vi "PSA E4440A Set and Read Marker X and Y Values.vi"(0 "VISA resource name":refnum<visa-resource-name>, 1 "Marker Type (1: Position)":u16(ring)=1 items=["Off", "Position", "Delta", "Band", "Span Pair"], 2 "Readout (0: Frequency)":u16(ring) items=["Frequency", "Time", "Inverse Time", "Period"], 5 "Active Marker (1: Marker1)":u16(ring)=1 items=["Marker1"=1, "Marker2"=2, "Marker3"=3, "Marker4"=4], 9 "Zero Span":bool, 11 "error in (no error)":errorcluster, 12 "Span [Hz]":dbl=5000000.0 format="%.3p", 13 "Center Frequency (Hz)":dbl=2000000000.0) -> (4 "VISA resource name out":refnum<visa-resource-name>, 6 "Marker X Position (Hz)":dbl, 8 "Y Amplitude (dBm)":dbl, 15 "error out":errorcluster)   [LabVIEW 2015]
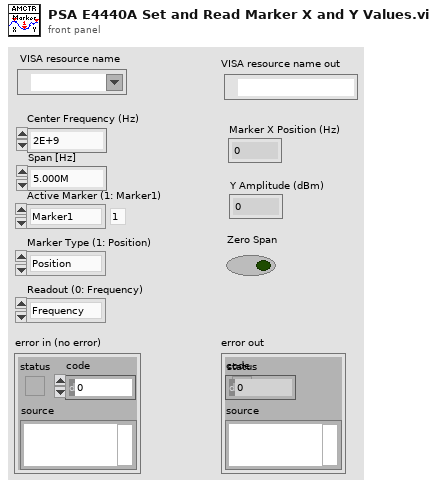
[diagram p1: front panel]
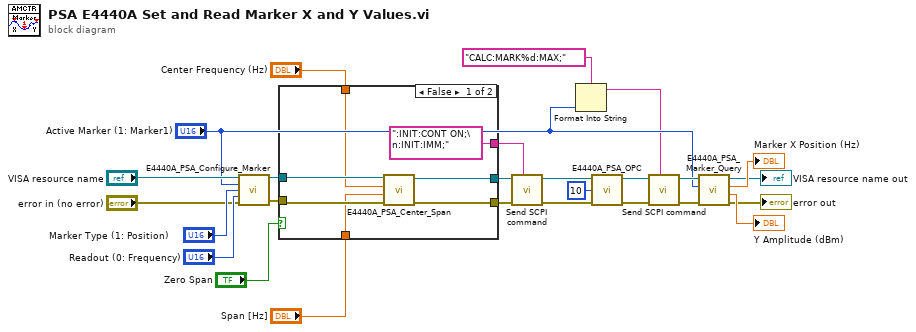
[diagram p0: block diagram]
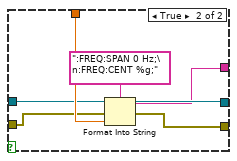
[diagram p2: hidden frame]
diagram:
  n1 = call "E4440A_PSA_Configure_Marker.vi"("VISA resource name"="VISA resource name", "Active Marker (1: Marker1)"="Active Marker (1: Marker1)", "Marker Type (1: Position)"="Marker Type (1: Position)", "Readout (0: Frequency)"="Readout (0: Frequency)", "error in (no error)"="error in (no error)") -> ("VISA resource name out"=w16:refnum<visa-resource-name>, "error out"=w17:errorcluster)  [unwired: 9 in]
  n2 = case shown="False" "Zero Span" {
    tunnel: [w33 w37] -> w22
    tunnel: [w32 w35] -> w21
    tunnel: w17 -> [w30 w36]
    tunnel: w16 -> [w31 w35]
    tunnel: "Center Frequency (Hz)" -> [w29 w38]
    tunnel: "Span [Hz]" -> [w28 _]
    tunnel: [":INIT:CONT ON;\n:INIT:IMM;" ("multi-line string") w34] -> w13
    frame False {
      n3 = call "E4440A_PSA_Center_Span.vi"("error in (no error)"=w30, "Span (2 GHz)"=w28, "Center Frequency (2 GHz)"=w29, "VISA resource name"=w31) -> ("error out"=w33:errorcluster, "VISA resource name out"=w32:refnum<visa-resource-name>)  [unwired: 6 in]
    }
    frame True {
      n4 = Format Into String(format string=":FREQ:SPAN 0 Hz;\n:FREQ:CENT %g;", error in=w36, w38) -> (resulting string=w34:string, error out=w37:errorcluster)  [unwired: 1 in]
    }
  }
  n5 = call "Send SCPI command.vi"("Send SCPI Command"=w13, "error in (no error)"=w22, "VISA resource name"=w21) -> ("error out"=w11:errorcluster, "VISA resource name out"=w10:refnum<visa-resource-name>)  [unwired: 7 in]
  n6 = Format Into String(format string="CALC:MARK%d:MAX;" ("Send SCPI Command"), "Active Marker (1: Marker1)") -> (resulting string=w1:string)  [unwired: 2 in, 1 out]
  n7 = call "E4440A_PSA_OPC.vi"("error in (no error)"=w11, "Wait (1000ms)"=u32 10, "VISA resource name"=w10) -> ("error out"=w7:errorcluster, "VISA resource name out"=w6:refnum<visa-resource-name>)  [unwired: 7 in]
  n8 = call "Send SCPI command.vi"("Send SCPI Command"=w1, "error in (no error)"=w7, "VISA resource name"=w6) -> ("error out"=w5:errorcluster, "VISA resource name out"=w4:refnum<visa-resource-name>)  [unwired: 7 in]
  n9 = call "E4440A_PSA_Marker_Query.vi"("error in (no error)"=w5, "Active Marker (1: Marker1)"="Active Marker (1: Marker1)", "VISA resource name"=w4) -> ("error out"=→"error out":errorcluster, "Marker Amplitude"=→"Y Amplitude (dBm)":dbl, "Marker Position"=→"Marker X Position (Hz)":dbl, "VISA resource name out"=→"VISA resource name out":refnum<visa-resource-name>)  [unwired: 5 in]
